vi "REPORT_get_number_of_pages.vi"(11 "rows":string[][](array[string])) -> (3 "nmb_of_pages":i32)   [LabVIEW 2019]
uses:
  FGV/main_ini/FGV_CLIENT_config_info.ctl
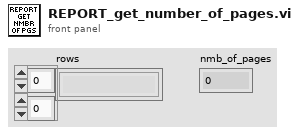
[diagram p1: front panel]
types:
  T1 = typedef "FGV_CLIENT_config_info.ctl" = enum16{"initialize", "set", "get"}
  T2 = typedef "CLIENT_all_config_info.ctl" = cluster{"main_ini_file":T3, "SQL Password":string, "queue_refnums":T4}
  T3 = typedef "CLIENT_main_ini_file.ctl" = cluster{"SQL Driver":string, "SQL Server":string, "SQL Database":string, "SQL UID":string, "Reference table":string, "Reference history":string, "Archivisation CFG table":string, "Archivisation CFG history":string, "User table":string, "User history":string, "logout timeout [ms]":i32, "records per page":i32, "default language":string, "REF CHG connection IP":string, "REF CHG remote port":i32, "REF CHG local port":i32, "SCANNER COM port":u16, "SCANNER Baud rate":u32, "SCANNER Data bits":u16, "SCANNER Pairity":enum16{"None", "Odd", "Even", "Mark", "Space"}, "SCANNER Stop bits":u16, "SCANNER Flow control":u16, "SCANNER Termination char":u8}
  T4 = typedef "CLIENT_queue_refnums.ctl" = cluster{"SQL_EDITOR_queue":refnum<queue>, "SCANNER_queue":refnum<queue>, "SCANNER_data":refnum<queue>, "CLIENT_REF_CHG_queue":refnum<queue>}
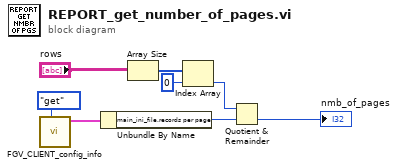
[diagram p0: block diagram]
diagram:
  n1 = call "FGV_CLIENT_config_info.vi"("options"=FGV_CLIENT_config_info."get") -> ("all_config_info_out"=w6:T2)  [unwired: 9 in, 1 out]
  n2 = Unbundle By Name(w6) -> ("main_ini_file.records per page"=w8:i32)
  n3 = Array Size(array="rows") -> (size(s)=w4:i32[])
  n4 = Index Array(array=w4, index=0) -> (element=w3:i32)
  n5 = Quotient & Remainder(x=w3, y=w8) -> (floor(x/y)=→"nmb_of_pages":i32)  [unwired: 1 out]
